vi "Calibration Convert String to Dates.vi"(8 "error in (no error)":errorcluster, 10 "all rows":string[](array[string]), 11 "Calibration Due in":T1 {"Eq20" format="%<%x>T"; "Eq19" format="%<%x>T"; "Eq18" format="%<%x>T"; "Eq17" format="%<%x>T"; "Eq16" format="%<%x>T"; "Eq15" format="%<%x>T"; "Eq14" format="%<%x>T"; "Eq13" format="%<%x>T"; "Eq12" format="%<%x>T"; "Eq11" format="%<%x>T"; "Eq10" format="%<%x>T"; "Eq9" format="%<%x>T"; "Eq8" format="%<%x>T"; "Eq7" format="%<%x>T"; "Eq6" format="%<%x>T"; "Eq5" format="%<%x>T"; "Eq4" format="%<%x>T"; "Eq3" format="%<%x>T"; "Eq2" format="%<%x>T"; "Eq1" format="%<%x>T"}) -> (0 "error out":errorcluster, 3 "Calibration Due out":T1 {"Eq20" format="%<%x>T"; "Eq19" format="%<%x>T"; "Eq18" format="%<%x>T"; "Eq17" format="%<%x>T"; "Eq16" format="%<%x>T"; "Eq15" format="%<%x>T"; "Eq14" format="%<%x>T"; "Eq13" format="%<%x>T"; "Eq12" format="%<%x>T"; "Eq11" format="%<%x>T"; "Eq10" format="%<%x>T"; "Eq9" format="%<%x>T"; "Eq8" format="%<%x>T"; "Eq7" format="%<%x>T"; "Eq6" format="%<%x>T"; "Eq5" format="%<%x>T"; "Eq4" format="%<%x>T"; "Eq3" format="%<%x>T"; "Eq2" format="%<%x>T"; "Eq1" format="%<%x>T"})   [LabVIEW 2020]
uses:
  Type Definitions/Calibration Time.ctl
panel:
  out "Array":i32[](array[numeric])
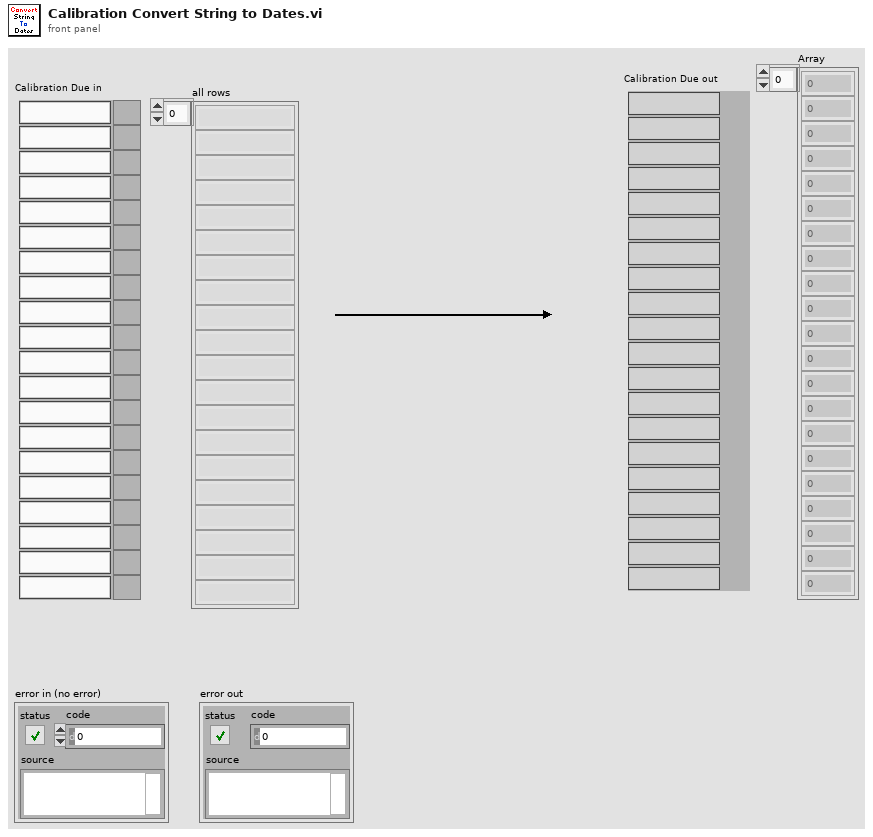
[diagram p1: front panel]
types:
  T1 = typedef "Calibration Time.ctl" = cluster{"Eq1":timestamp, "Eq2":timestamp, "Eq3":timestamp, "Eq4":timestamp, "Eq5":timestamp, "Eq6":timestamp, "Eq7":timestamp, "Eq8":timestamp, "Eq9":timestamp, "Eq10":timestamp, "Eq11":timestamp, "Eq12":timestamp, "Eq13":timestamp, "Eq14":timestamp, "Eq15":timestamp, "Eq16":timestamp, "Eq17":timestamp, "Eq18":timestamp, "Eq19":timestamp, "Eq20":timestamp}
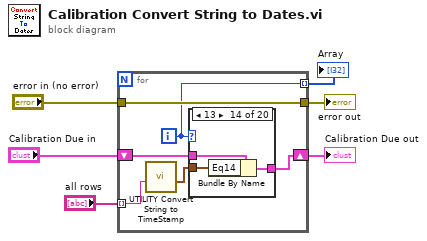
[diagram p0: block diagram]
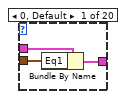
[diagram p2: hidden frame]
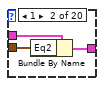
[diagram p3: hidden frame]
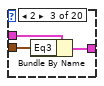
[diagram p4: hidden frame]
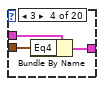
[diagram p5: hidden frame]
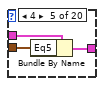
[diagram p6: hidden frame]
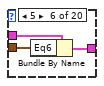
[diagram p7: hidden frame]
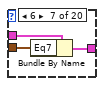
[diagram p8: hidden frame]
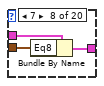
[diagram p9: hidden frame]
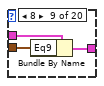
[diagram p10: hidden frame]
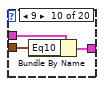
[diagram p11: hidden frame]
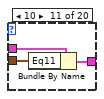
[diagram p12: hidden frame]
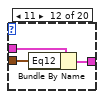
[diagram p13: hidden frame]
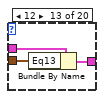
[diagram p14: hidden frame]
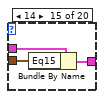
[diagram p15: hidden frame]
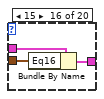
[diagram p16: hidden frame]
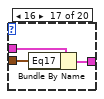
[diagram p17: hidden frame]
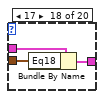
[diagram p18: hidden frame]
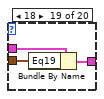
[diagram p19: hidden frame]
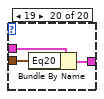
[diagram p20: hidden frame]
diagram:
  n1 = for {
    tunnel: "all rows" -> [w12] mode=indexing
    shift-right: [w9] -> w5
    shift-left: "Calibration Due in" -> [w11]
    tunnel: [w8] -> w4
    tunnel: "error in (no error)" -> [w8]
    tunnel: [w7] -> w1 mode=indexing
    i -> [w7]
    n2 = call "UTILITY Convert String to TimeStamp.vi"("Date"=w12) -> ("Resulting Date Stamp"=w10:timestamp)  [unwired: 9 in, 1 out]
    n3 = case shown="13" w7 {
      tunnel: w11 -> [w14 w17 w20 w23 w26 w29 w32 w35 w38 w41 w44 w47 w50 w53 w57 w60 w63 w66 w68 w71]
      tunnel: w10 -> [w15 w18 w21 w24 w27 w30 w33 w36 w39 w42 w45 w48 w51 w54 w56 w59 w62 w64 w69 w72]
      tunnel: [w13 w16 w19 w22 w25 w28 w31 w34 w37 w40 w43 w46 w49 w52 w55 w58 w61 w65 w67 w70] -> w9
      frame 0, Default {
        n4 = Bundle By Name(cluster=w14, "Eq1"=w15) -> (w13:T1)
      }
      frame 1 {
        n5 = Bundle By Name(cluster=w17, "Eq2"=w18) -> (w16:T1)
      }
      frame 2 {
        n6 = Bundle By Name(cluster=w20, "Eq3"=w21) -> (w19:T1)
      }
      frame 3 {
        n7 = Bundle By Name(cluster=w23, "Eq4"=w24) -> (w22:T1)
      }
      frame 4 {
        n8 = Bundle By Name(cluster=w26, "Eq5"=w27) -> (w25:T1)
      }
      frame 5 {
        n9 = Bundle By Name(cluster=w29, "Eq6"=w30) -> (w28:T1)
      }
      frame 6 {
        n10 = Bundle By Name(cluster=w32, "Eq7"=w33) -> (w31:T1)
      }
      frame 7 {
        n11 = Bundle By Name(cluster=w35, "Eq8"=w36) -> (w34:T1)
      }
      frame 8 {
        n12 = Bundle By Name(cluster=w38, "Eq9"=w39) -> (w37:T1)
      }
      frame 9 {
        n13 = Bundle By Name(cluster=w41, "Eq10"=w42) -> (w40:T1)
      }
      frame 10 {
        n14 = Bundle By Name(cluster=w44, "Eq11"=w45) -> (w43:T1)
      }
      frame 11 {
        n15 = Bundle By Name(cluster=w47, "Eq12"=w48) -> (w46:T1)
      }
      frame 12 {
        n16 = Bundle By Name(cluster=w50, "Eq13"=w51) -> (w49:T1)
      }
      frame 13 {
        n17 = Bundle By Name(cluster=w53, "Eq14"=w54) -> (w52:T1)
      }
      frame 14 {
        n18 = Bundle By Name(cluster=w57, "Eq15"=w56) -> (w55:T1)
      }
      frame 15 {
        n19 = Bundle By Name(cluster=w60, "Eq16"=w59) -> (w58:T1)
      }
      frame 16 {
        n20 = Bundle By Name(cluster=w63, "Eq17"=w62) -> (w61:T1)
      }
      frame 17 {
        n21 = Bundle By Name(cluster=w66, "Eq18"=w64) -> (w65:T1)
      }
      frame 18 {
        n22 = Bundle By Name(cluster=w68, "Eq19"=w69) -> (w67:T1)
      }
      frame 19 {
        n23 = Bundle By Name(cluster=w71, "Eq20"=w72) -> (w70:T1)
      }
    }
  }
  "Calibration Due out" <- w5
  "error out" <- w4
  "Array" <- w1
